vi "Handle Stabilization.vi"(0 "DesiredCluster":T2, 1 "Controller?":bool, 2 "AveFeedback":dbl[](array[numeric]), 7 "Tolerances":dbl[](array[numeric]), 9 "AveControllerCMD":dbl format="%#_13g", 11 "StabilityCluster In":T1) -> (4 "BoundsArray":dbl[][](array[numeric]), 8 "StableArray":bool[](array[boolean]), 15 "StabilityCluster Out":T1)   [LabVIEW 2013]
uses:
  TypeDef/Command Cluster.ctl
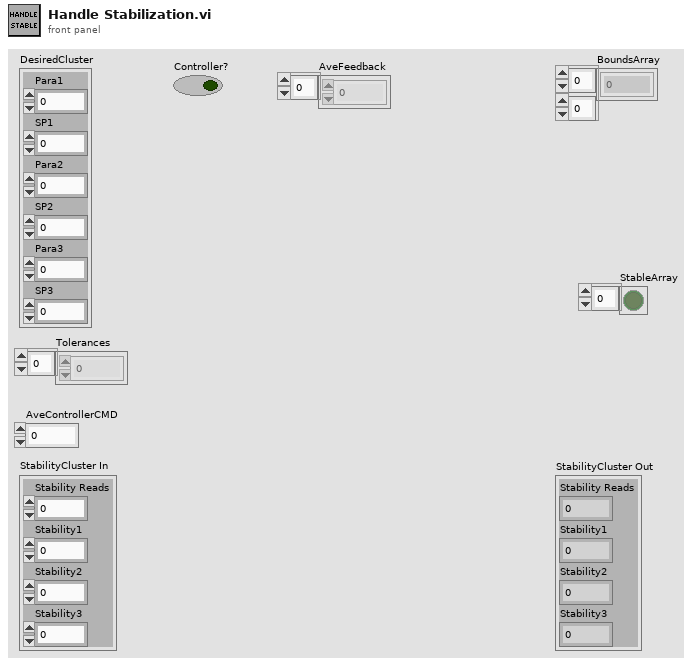
[diagram p1: front panel]
types:
  T1 = cluster{"Stability Reads":i32, "Stability1":i32, "Stability2":i32, "Stability3":i32}
  T2 = typedef "Command Cluster.ctl" = cluster{"Para1":i32, "SP1":dbl, "Para2":i32, "SP2":dbl, "Para3":i32, "SP3":dbl}
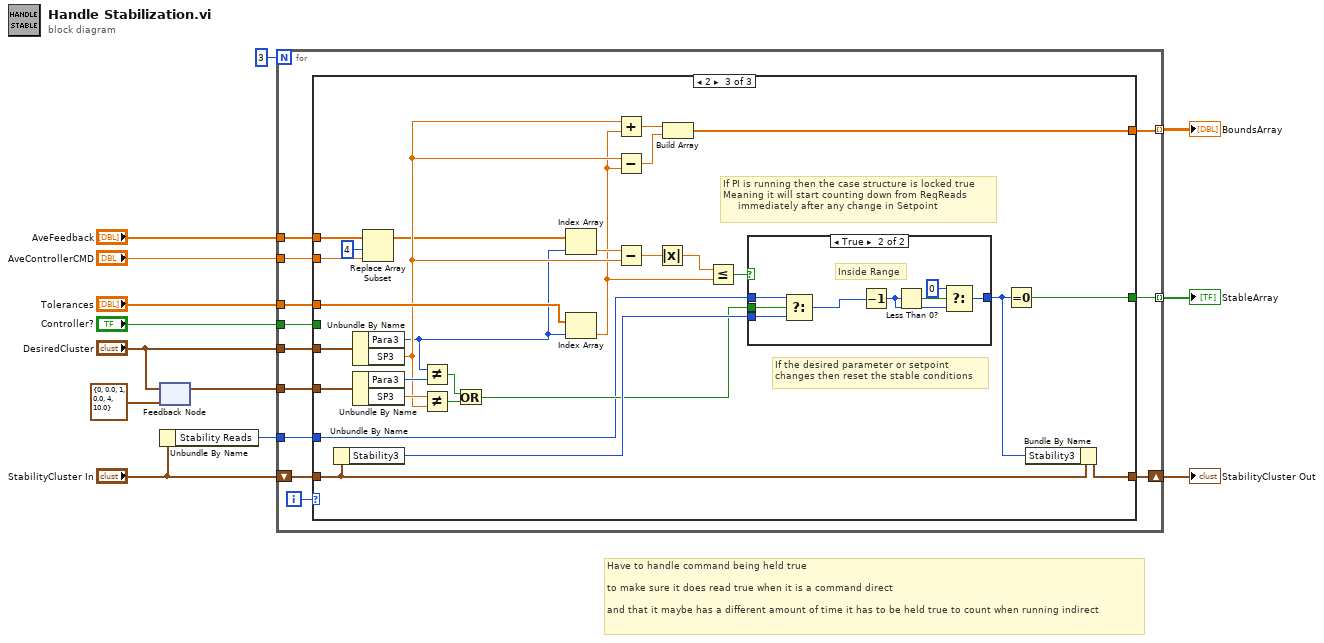
[diagram p0: block diagram]
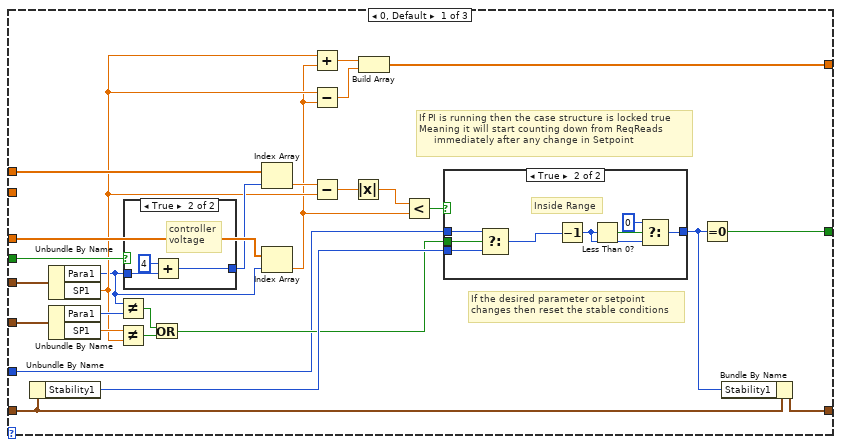
[diagram p2: hidden frame]
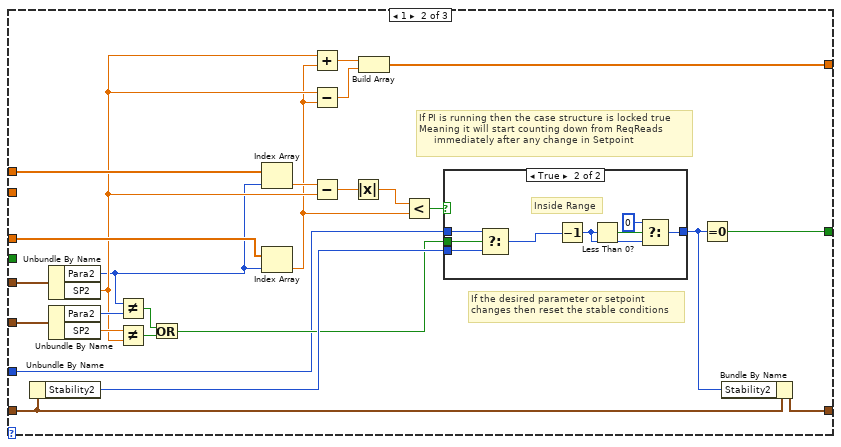
[diagram p5: hidden frame]
diagram:
  # "Have to handle command being held true\n\nto make sure it does read true when it is a command direct\n\nand that it maybe has a different amount of time it has to be held true to count when running indirect"
  n1 = feedback-in #1("DesiredCluster") -> ()
  n2 = feedback #1(T2 {"Para1"=0, "SP1"=0.0, "Para2"=1, "SP2"=0.0, "Para3"=4, "SP3"=10.0} ("DesiredCluster")) -> (w6:T2)
  n3 = Unbundle By Name("StabilityCluster In") -> ("Stability Reads"=w12:i32)
  n4 = for {
    N: 3 -> [_]
    shift-right: [w21] -> w2
    shift-left: "StabilityCluster In" -> [w23]
    tunnel: w12 -> [w24]
    tunnel: "DesiredCluster" -> [w22]
    tunnel: "AveFeedback" -> [w19]
    tunnel: "Tolerances" -> [w20]
    tunnel: "Controller?" -> [w18]
    tunnel: w6 -> [w17]
    tunnel: [w16] -> w5 mode=indexing
    tunnel: [w15] -> w4 mode=indexing
    tunnel: "AveControllerCMD" -> [w14]
    i -> [w25]
    n5 = case shown="2" w25 {
      tunnel: w24 -> [w39 w78 w115]
      tunnel: w23 -> [w50 w89 w126]
      tunnel: w22 -> [w52 w90 w127]
      tunnel: [w49 w88 w125] -> w21
      tunnel: w20 -> [w48 w87 w124]
      tunnel: w19 -> [w38 w77 w101]
      tunnel: w18 -> [w51 _ _]
      tunnel: w17 -> [w47 w86 w123]
      tunnel: [w29 w69 w107] -> w16
      tunnel: [w28 w68 w106] -> w15
      tunnel: w14 -> [_ _ w103]
      frame 0, Default {
        # "If PI is running then the case structure is locked true\nMeaning it will start counting down from ReqReads\n     immediately after any change in Setpoint"
        # "If the desired parameter or setpoint\nchanges then reset the stable conditions"
        n6 = Unbundle By Name(w50) -> ("Stability1"=w42:i32)
        n7 = Unbundle By Name(w52) -> ("Para1"=w26:i32, "SP1"=w33:dbl)
        n8 = Unbundle By Name(w47) -> ("Para1"=w46:i32, "SP1"=w45:dbl)
        n9 = Not Equal?(x=w26, y=w46) -> (x != y?=w44:bool)
        n10 = Not Equal?(x=w45, y=w33) -> (x != y?=w43:bool)
        n11 = case shown="True" w51 {
          tunnel: w26 -> [w62 w65]
          tunnel: [w62 w63] -> w37
          frame False {
            # "pump\nvoltage"
          }
          frame True {
            # "controller\nvoltage"
            n12 = Add(x=4, y=w65) -> (x+y=w63:i32)
          }
        }
        n13 = Or(x=w44, y=w43) -> (x .or. y?=w40:bool)
        n14 = Index Array(array=w38, index=w37) -> (element=w36:dbl)
        n15 = Index Array(array=w48, index=w26) -> (element=w32:dbl)
        n16 = Add(x=w33, y=w32) -> (x+y=w31:dbl)
        n17 = Subtract(x=w33, y=w32) -> (x-y=w30:dbl)
        n18 = Subtract(x=w36, y=w33) -> (x-y=w35:dbl)
        n19 = Absolute Value(x=w35) -> (abs(x)=w34:dbl)
        n20 = Build Array(w31, w30) -> (w29:dbl[])
        n21 = Less?(x=w34, y=w32) -> (x < y?=w27:bool)
        n22 = case shown="True" w27 {
          tunnel: [w53 w58] -> w41
          tunnel: w39 -> [w53 w56]
          tunnel: w40 -> [_ w57]
          tunnel: w42 -> [_ w54]
          frame False {
            # "Outside Range"
          }
          frame True {
            # "Inside Range"
            n23 = Select(t=w56, s=w57, f=w54) -> (s? t:f=w55:i32)
            n24 = Decrement(x=w55) -> (x-1=w60:i32)
            n25 = Less Than 0?(x=w60) -> (x < 0?=w59:bool)
            n26 = Select(t=0, s=w59, f=w60) -> (s? t:f=w58:i32)
          }
        }
        n27 = Equal To 0?(x=w41) -> (x = 0?=w28:bool)
        n28 = Bundle By Name(cluster=w50, "Stability1"=w41) -> (w49:T1)
      }
      frame 1 {
        # "If PI is running then the case structure is locked true\nMeaning it will start counting down from ReqReads\n     immediately after any change in Setpoint"
        # "If the desired parameter or setpoint\nchanges then reset the stable conditions"
        n29 = Unbundle By Name(w89) -> ("Stability2"=w81:i32)
        n30 = Unbundle By Name(w90) -> ("Para2"=w66:i32, "SP2"=w73:dbl)
        n31 = Unbundle By Name(w86) -> ("Para2"=w85:i32, "SP2"=w84:dbl)
        n32 = Not Equal?(x=w66, y=w85) -> (x != y?=w83:bool)
        n33 = Not Equal?(x=w84, y=w73) -> (x != y?=w82:bool)
        n34 = Or(x=w83, y=w82) -> (x .or. y?=w79:bool)
        n35 = Index Array(array=w77, index=w66) -> (element=w76:dbl)
        n36 = Index Array(array=w87, index=w66) -> (element=w72:dbl)
        n37 = Add(x=w73, y=w72) -> (x+y=w71:dbl)
        n38 = Subtract(x=w73, y=w72) -> (x-y=w70:dbl)
        n39 = Subtract(x=w76, y=w73) -> (x-y=w75:dbl)
        n40 = Absolute Value(x=w75) -> (abs(x)=w74:dbl)
        n41 = Build Array(w71, w70) -> (w69:dbl[])
        n42 = Less?(x=w74, y=w72) -> (x < y?=w67:bool)
        n43 = case shown="True" w67 {
          tunnel: [w91 w96] -> w80
          tunnel: w78 -> [w91 w94]
          tunnel: w79 -> [_ w95]
          tunnel: w81 -> [_ w92]
          frame False {
            # "Outside Range"
          }
          frame True {
            # "Inside Range"
            n44 = Select(t=w94, s=w95, f=w92) -> (s? t:f=w93:i32)
            n45 = Decrement(x=w93) -> (x-1=w98:i32)
            n46 = Less Than 0?(x=w98) -> (x < 0?=w97:bool)
            n47 = Select(t=0, s=w97, f=w98) -> (s? t:f=w96:i32)
          }
        }
        n48 = Equal To 0?(x=w80) -> (x = 0?=w68:bool)
        n49 = Bundle By Name(cluster=w89, "Stability2"=w80) -> (w88:T1)
      }
      frame 2 {
        # "If PI is running then the case structure is locked true\nMeaning it will start counting down from ReqReads\n     immediately after any change in Setpoint"
        # "If the desired parameter or setpoint\nchanges then reset the stable conditions"
        n50 = Unbundle By Name(w126) -> ("Stability3"=w118:i32)
        n51 = Unbundle By Name(w127) -> ("Para3"=w104:i32, "SP3"=w111:dbl)
        n52 = Unbundle By Name(w123) -> ("Para3"=w122:i32, "SP3"=w121:dbl)
        n53 = Replace Array Subset(array=w101, new element=w103, index=4) -> (w100:dbl[])
        n54 = Not Equal?(x=w104, y=w122) -> (x != y?=w120:bool)
        n55 = Not Equal?(x=w121, y=w111) -> (x != y?=w119:bool)
        n56 = Or(x=w120, y=w119) -> (x .or. y?=w116:bool)
        n57 = Index Array(array=w100, index=w104) -> (element=w114:dbl)
        n58 = Index Array(array=w124, index=w104) -> (element=w110:dbl)
        n59 = Add(x=w111, y=w110) -> (x+y=w109:dbl)
        n60 = Subtract(x=w111, y=w110) -> (x-y=w108:dbl)
        n61 = Subtract(x=w114, y=w111) -> (x-y=w113:dbl)
        n62 = Absolute Value(x=w113) -> (abs(x)=w112:dbl)
        n63 = Build Array(w109, w108) -> (w107:dbl[])
        n64 = Less Or Equal?(x=w112, y=w110) -> (x <= y?=w105:bool)
        n65 = case shown="True" w105 {
          tunnel: [w128 w133] -> w117
          tunnel: w115 -> [w128 w131]
          tunnel: w116 -> [_ w132]
          tunnel: w118 -> [_ w129]
          frame False {
            # "Outside Range"
          }
          frame True {
            # "Inside Range"
            n66 = Select(t=w131, s=w132, f=w129) -> (s? t:f=w130:i32)
            n67 = Decrement(x=w130) -> (x-1=w135:i32)
            n68 = Less Than 0?(x=w135) -> (x < 0?=w134:bool)
            n69 = Select(t=0, s=w134, f=w135) -> (s? t:f=w133:i32)
          }
        }
        n70 = Equal To 0?(x=w117) -> (x = 0?=w106:bool)
        n71 = Bundle By Name(cluster=w126, "Stability3"=w117) -> (w125:T1)
      }
    }
  }
  "BoundsArray" <- w5
  "StableArray" <- w4
  "StabilityCluster Out" <- w2
